vi "3.6.vi"() -> ()   [LabVIEW 2014]
panel:
  in  "CONVERTION":T1(ring)
  in  "?":bool
  out "END TEMP":dbl
  in  "START TEMP":dbl
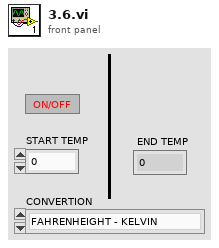
[diagram p1: front panel]
types:
  T1 = enum16{"FAHRENHEIGHT - KELVIN", "CELCIUS - KELVIN", "FAHRENHEIGHT - CELCIUS", "CELCIUS - FAHRENHEIGHT"}
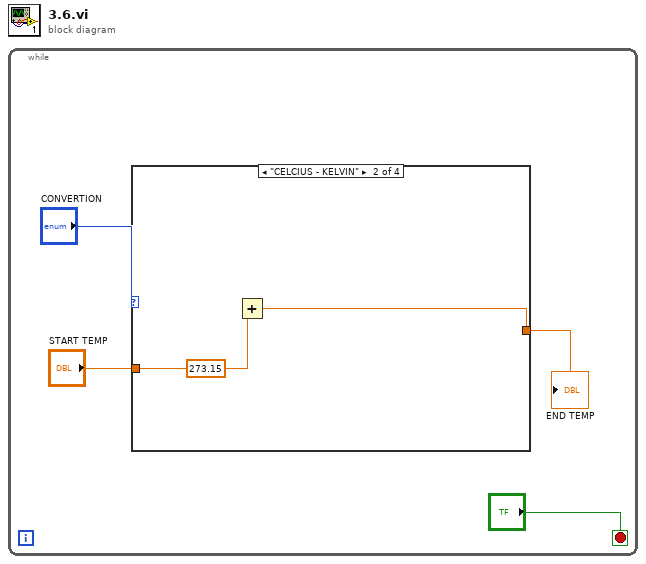
[diagram p0: block diagram]
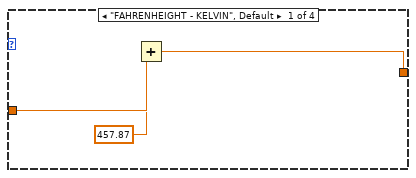
[diagram p2: hidden frame]
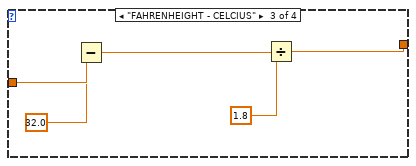
[diagram p3: hidden frame]
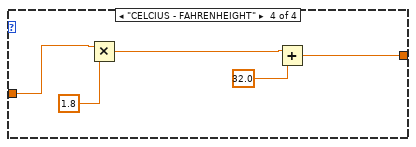
[diagram p4: hidden frame]
diagram:
  n1 = while {
    stop <- "?" stop-if-true
    n2 = case shown="\"CELCIUS - KELVIN\"" "CONVERTION" {
      tunnel: "START TEMP" -> [w7 w9 w15 w19]
      tunnel: [w5 w8 w11 w16] -> w1
      frame "FAHRENHEIGHT - KELVIN", Default {
        n3 = Add(x=w7, y=457.87) -> (x+y=w5:dbl)
      }
      frame "CELCIUS - KELVIN" {
        n4 = Add(x=w9, y=273.15) -> (x+y=w8:dbl)
      }
      frame "FAHRENHEIGHT - CELCIUS" {
        n5 = Subtract(x=w15, y=32.0) -> (x-y=w13:dbl)
        n6 = Divide(x=w13, y=1.8) -> (x/y=w11:dbl)
      }
      frame "CELCIUS - FAHRENHEIGHT" {
        n7 = Multiply(x=w19, y=1.8) -> (x*y=w18:dbl)
        n8 = Add(x=w18, y=32.0) -> (x+y=w16:dbl)
      }
    }
    "END TEMP" <- w1
  }
